vi "Start Free-Run.vi"(8 "error in (no error)":errorcluster, 10 "Measurement (0: Level)":i32(ring) items=["Level", "SNR", "THDN", "Distortion", "IMDistortion", "Crosstalk", "FrequencyResponse", "InputOutputPhase", "InterchannelPhase"], 11 "VISA resource name":refnum<visa-resource-name>) -> (0 "error out":errorcluster, 3 "VISA resource name out":refnum<visa-resource-name>)   [LabVIEW 2014, in "Stanford Research SR1.lvlib"]
doc: "Starts the free-run for the selected measurement."
uses:
  Stanford Research SR1.lvlib
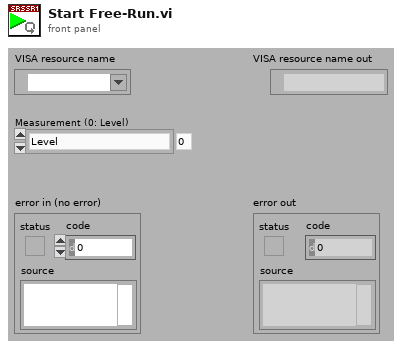
[diagram p1: front panel]
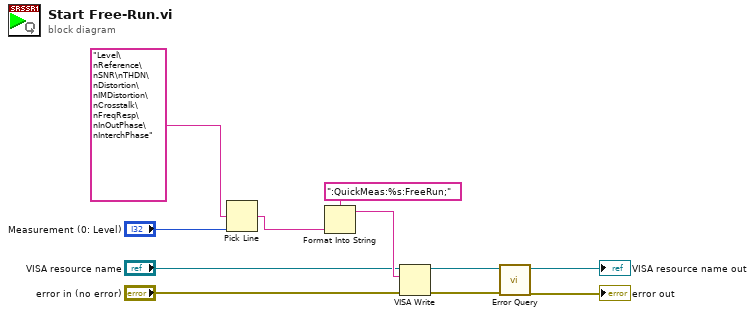
[diagram p0: block diagram]
diagram:
  n1 = Pick Line(multi-line string="Level\nReference\nSNR\nTHDN\nDistortion\nIMDistortion\nCrosstalk\nFreqResp\nInOutPhase\nInterchPhase", line index="Measurement (0: Level)") -> (output string=w1:string)  [unwired: 1 in]
  n2 = Format Into String(format string=":QuickMeas:%s:FreeRun;", w1) -> (resulting string=w10:string)  [unwired: 2 in, 1 out]
  n3 = VISA Write(VISA resource name="VISA resource name", write buffer=w10, error in (no error)="error in (no error)") -> (VISA resource name out=w7:refnum<visa-resource-name>, error out=w6:errorcluster)  [unwired: 1 out]
  n4 = call "Error Query.vi"("error in (no error)"=w6, "VISA resource name"=w7) -> ("error out"=→"error out":errorcluster, "VISA resource name out"=→"VISA resource name out":refnum<visa-resource-name>)  [unwired: 6 in, 2 out]
